vi "Pause.vi"(7 "timeout in ms (-1)":i32=-1, 8 "error in (no error)":errorcluster, 11 "index":i32) -> (0 "error out":errorcluster)   [LabVIEW 2019, in "Unit Test Engine Tools.lvlib"]
uses:
  Unit Test Engine Tools.lvlib
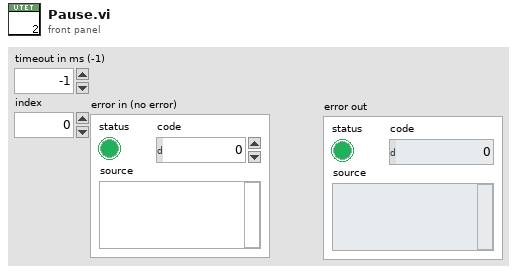
[diagram p1: front panel]
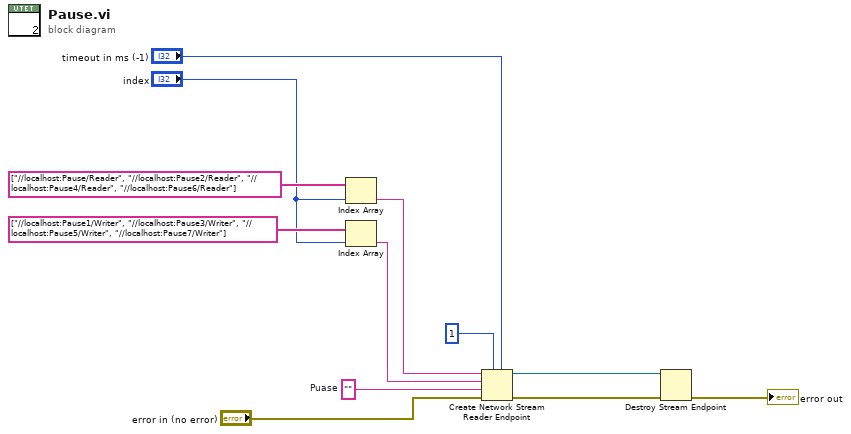
[diagram p0: block diagram]
diagram:
  w9 = ""  # Puase
  n1 = Index Array(array=string[] ["//localhost:Pause/Reader", "//localhost:Pause2/Reader", "//localhost:Pause4/Reader", "//localhost:Pause6/Reader"], index="index") -> (element=w1:string)
  n2 = Index Array(array=string[] ["//localhost:Pause1/Writer", "//localhost:Pause3/Writer", "//localhost:Pause5/Writer", "//localhost:Pause7/Writer"], index="index") -> (element=w2:string)
  n3 = Create Network Stream Reader Endpoint(5:"timeout in ms (-1)", 7:1 ("reader buffer size"), 8:"error in (no error)", 9:w9, 10:w2, 11:w1) -> (0:w7:errorcluster, 3:w8:refnum<k21>)  [unwired: 1 in]
  n4 = Destroy Stream Endpoint(8:w7, 11:w8) -> (0:→"error out":errorcluster)
